vi "Target.vi"() -> ()   [LabVIEW 2018]
uses:
  <vilib>/Platform/TimedLoop/XDataNode/timing_clust.ctl
  <vilib>/Platform/TimedLoop/XDataNode/nitl_modes.ctl
  <vilib>/Platform/TimedLoop/XDataNode/wakeup.ctl
  <vilib>/rvi/eio/common/nirviEmuTemplateMethod_errors.vi
  <vilib>/rvi/Emulation/niFpgaGetClockAttributes.vi
  <vilib>/rvi/Emulation/niFpgaSctlEmulationGetInTimedLoop.vi
  <vilib>/rvi/Emulation/niFpgaEmulationReportErrorSimple.vi
  <vilib>/rvi/Emulation/niFpgaProcessEmulError.vi
  <vilib>/rvi/Emulation/niFpgaCriticalErrorInLSC.vi
  <vilib>/rvi/DataTransferAndStorage/Container/Common/niFpgaContainerGetUniqueNameForEmu.vi
  <vilib>/rvi/Memory/Memory_Emulation/niFpgaMemoryFastEmulationDramWriteAndRequestData.vi
  <vilib>/rvi/Memory/Memory_Emulation/niFpgaMemoryEmulationDramWriteAndRequestData.vi
  <vilib>/rvi/Memory/Memory_Emulation/niFpgaMemoryEmulationDramWriteAndRequestDataApplyByteEnables.vi
  <vilib>/rvi/interface/RandomDataEmulation/niFpgaRandomDataHandleErrors.vi
  <vilib>/eio/EIONode/EIONode.xnode
  <vilib>/Platform/TimedLoop/XDataNode/XDataNode.xnode
  <vilib>/rvi/DataTransferAndStorage/Container/XNode/niFpgaContainer.xnode
  <vilib>/rvi/Memory/Memory_Emulation/niFpgaMemoryEmulationDramRetrieveData.vi
  <vilib>/rvi/interface/RandomDataEmulation/nirviRandomDataFpgaReadWriteTemplate.vi
  <vilib>/Platform/TimedLoop/XDataNode/XDNodeRunTimeDep.lvlib
panel:
  in  "SYNC":bool
  in  "Top(T)/Bot(F)":bool
  in  "SPI_532":u16=532
  in  "SPI_260":u16=260
  in  "W(T)/R(F)":bool
  in  "SPI_258":u16=258
  in  "SPI_256":u16=256
  in  "SPI_257":u16=257
  in  "472":u16=472
  in  "477":u16=477
  in  "478":u16=478
  in  "482":u16=482
  in  "500":u16=500
  in  "503":u16=503
  in  "540":u16=540
  in  "558":u16=558
  in  "559":u16=559
  in  "280":u16=280
  in  "348":u16=348
  in  "351":u16=351
  in  "352":u16=352
  in  "355":u16=355
  in  "357":u16=357
  in  "394":u16=394
  in  "399":u16=399
  in  "400":u16=400
  in  "470":u16=470
  in  "134":u16=134
  in  "140":u16=140
  in  "180":u16=180
  in  "220":u16=220
  in  "222":u16=222
  in  "223":u16=223
  in  "224":u16=224
  in  "225":u16=225
  in  "274":u16=274
  in  "279":u16=279
  in  "75":u16=75
  in  "100":u16=100
  in  "107":u16=107
  in  "109":u16=109
  in  "120":u16=120
  in  "121":u16=121
  in  "124":u16=124
  in  "125":u16=125
  in  "128":u16=128
  in  "130":u16=130
  in  "39":u16=39
  in  "33":u16=33
  in  "30":u16=30
  in  "29":u16=29
  in  "28":u16=28
  in  "26":u16=26
  in  "18":u16=18
  in  "15":u16=15
  in  "12":u16=12
  in  "Управление":bool
  in  "560":u16=560
  in  "12_CLK":u8=12
  in  "DATA_16":u8=16
  in  "6881280":u32=6881280
  in  "Стоп":bool
  out "SPI_OFF":bool
  in  "SPI_IN":bool[](array[boolean])
  out "SPI_OUT":bool[](array[boolean])=[FALSE, FALSE, FALSE, FALSE, FALSE, FALSE, FALSE, FALSE, FALSE, FALSE, FALSE, FALSE, FALSE, FALSE, FALSE, FALSE, FALSE, FALSE, FALSE, FALSE, FALSE, FALSE, FALSE, FALSE, FALSE, FALSE, FALSE, FALSE, FALSE, TRUE, FALSE, TRUE, FALSE, TRUE, FALSE, TRUE, TRUE, TRUE, FALSE, FALSE, TRUE, FALSE, TRUE, TRUE, FALSE, FALSE, FALSE, TRUE, TRUE, TRUE, TRUE, FALSE, FALSE, FALSE, FALSE, FALSE, TRUE, TRUE, TRUE, FALSE, FALSE, FALSE, FALSE, TRUE, TRUE, FALSE, FALSE, FALSE, FALSE, FALSE, FALSE, TRUE, TRUE, FALSE, TRUE, FALSE, TRUE, TRUE, TRUE, FALSE, TRUE, FALSE, TRUE, FALSE, FALSE, FALSE, TRUE, FALSE, FALSE, TRUE, TRUE, FALSE, FALSE, TRUE, TRUE, FALSE, FALSE, FALSE, FALSE, FALSE, FALSE, TRUE, TRUE, TRUE, FALSE, TRUE, TRUE, FALSE, FALSE, TRUE, FALSE, FALSE, FALSE, TRUE, TRUE, FALSE, TRUE, TRUE, FALSE, TRUE, FALSE, FALSE, TRUE, TRUE, TRUE, TRUE, TRUE, TRUE, TRUE, FALSE, TRUE, FALSE, FALSE, TRUE, TRUE, FALSE, FALSE, TRUE, FALSE, FALSE, FALSE, FALSE, TRUE, TRUE, TRUE, FALSE, TRUE, FALSE, FALSE, TRUE, FALSE, TRUE, TRUE, FALSE, TRUE, TRUE, TRUE, FALSE, TRUE, FALSE, TRUE, FALSE, TRUE, TRUE, FALSE, FALSE, TRUE, TRUE, FALSE, TRUE, TRUE, TRUE, TRUE, TRUE, TRUE, TRUE, FALSE, TRUE, TRUE, FALSE, TRUE, FALSE, TRUE, FALSE, TRUE, FALSE, TRUE, FALSE, FALSE, FALSE, FALSE, TRUE, FALSE, FALSE, FALSE, TRUE, FALSE, FALSE, FALSE, TRUE, FALSE, FALSE, TRUE, TRUE, TRUE, TRUE, TRUE, FALSE, FALSE, TRUE, FALSE, FALSE, FALSE, TRUE, TRUE, TRUE, TRUE, FALSE, TRUE, TRUE, TRUE, FALSE, FALSE, TRUE, TRUE, TRUE, TRUE, TRUE, FALSE, TRUE, TRUE, TRUE, FALSE, TRUE, FALSE, FALSE, FALSE, TRUE, FALSE, FALSE, TRUE, FALSE, FALSE, FALSE, FALSE, FALSE, TRUE, TRUE, FALSE, FALSE, TRUE, FALSE, TRUE, FALSE, FALSE, FALSE, FALSE, TRUE, FALSE, FALSE, FALSE, TRUE, FALSE, TRUE, TRUE, FALSE, TRUE, TRUE, FALSE, TRUE, TRUE, TRUE]
  in  "SPI":bool
  in  "SYS_RESET":bool
  in  "Автомат":bool
  out "Записали адресов":u32
  in  "Кадр в память":bool
  in  "Кадр на ПК":bool
  in  "Нач_адр":u32
  in  "Кон_адр":u32=122880
  out "Записали FIFO":bool
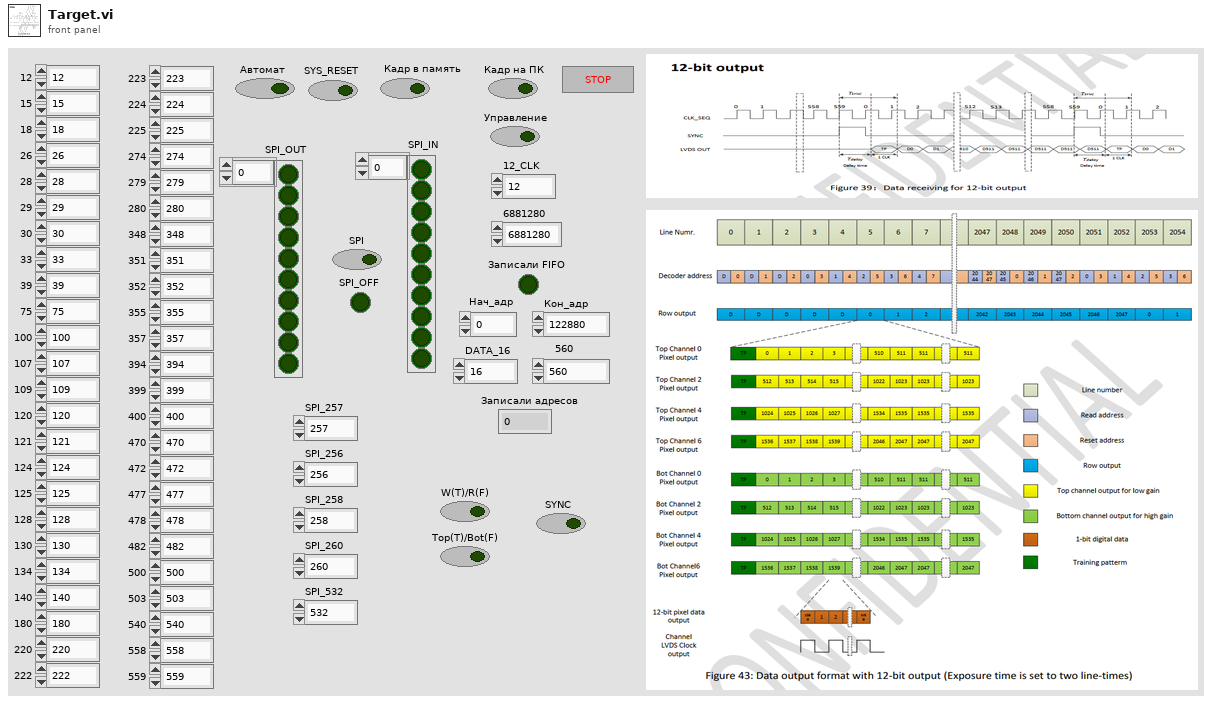
[diagram p1: front panel]
types:
  T1 = typedef "XDNodeRunTimeDep.lvlib/timing_clust.ctl" = cluster{"Expected End [f-1]":u64, "Actual End [f-1]":u64, "Finished Late? [f-1]":bool, "Expected End [i-1]":u64, "Actual End [i-1]":u64, "Finished Late? [i-1]":bool, "Expected Start [i]":u64, "Actual Start [i]":u64, "Expected Start [f]":u64, "Actual Start [f]":u64, "Source Name":string, "Structure Name":string, "Period":i64, "Deadline":i64, "Offset":i64, "Start":i64, "Priority":i32, "Timeout":i32, "Mode":T2, "Wakeup Reason":T3, "Error":errorcluster, "Source Type":string, "Secondary Source Type":string, "Global End Time":u64, "Global Start Time":u64, "Frame Duration":u64, "Iteration Duration":u64, "Assigned CPU":i32, "I/O Scan Engine Mode":u32}
  T2 = typedef "XDNodeRunTimeDep.lvlib/nitl_modes.ctl" = enum32{"No Change", "Process missed periods, maintain original phase", "Discard missed periods, maintain original phase", "Process missed periods, ignore original phase", "Discard missed periods, ignore original phase"}
  T3 = typedef "XDNodeRunTimeDep.lvlib/wakeup.ctl" = enum32{"Normal", "Aborted", "Asynchronous wakeup", "Timing source error", "Timed loop error", "Timeout"}
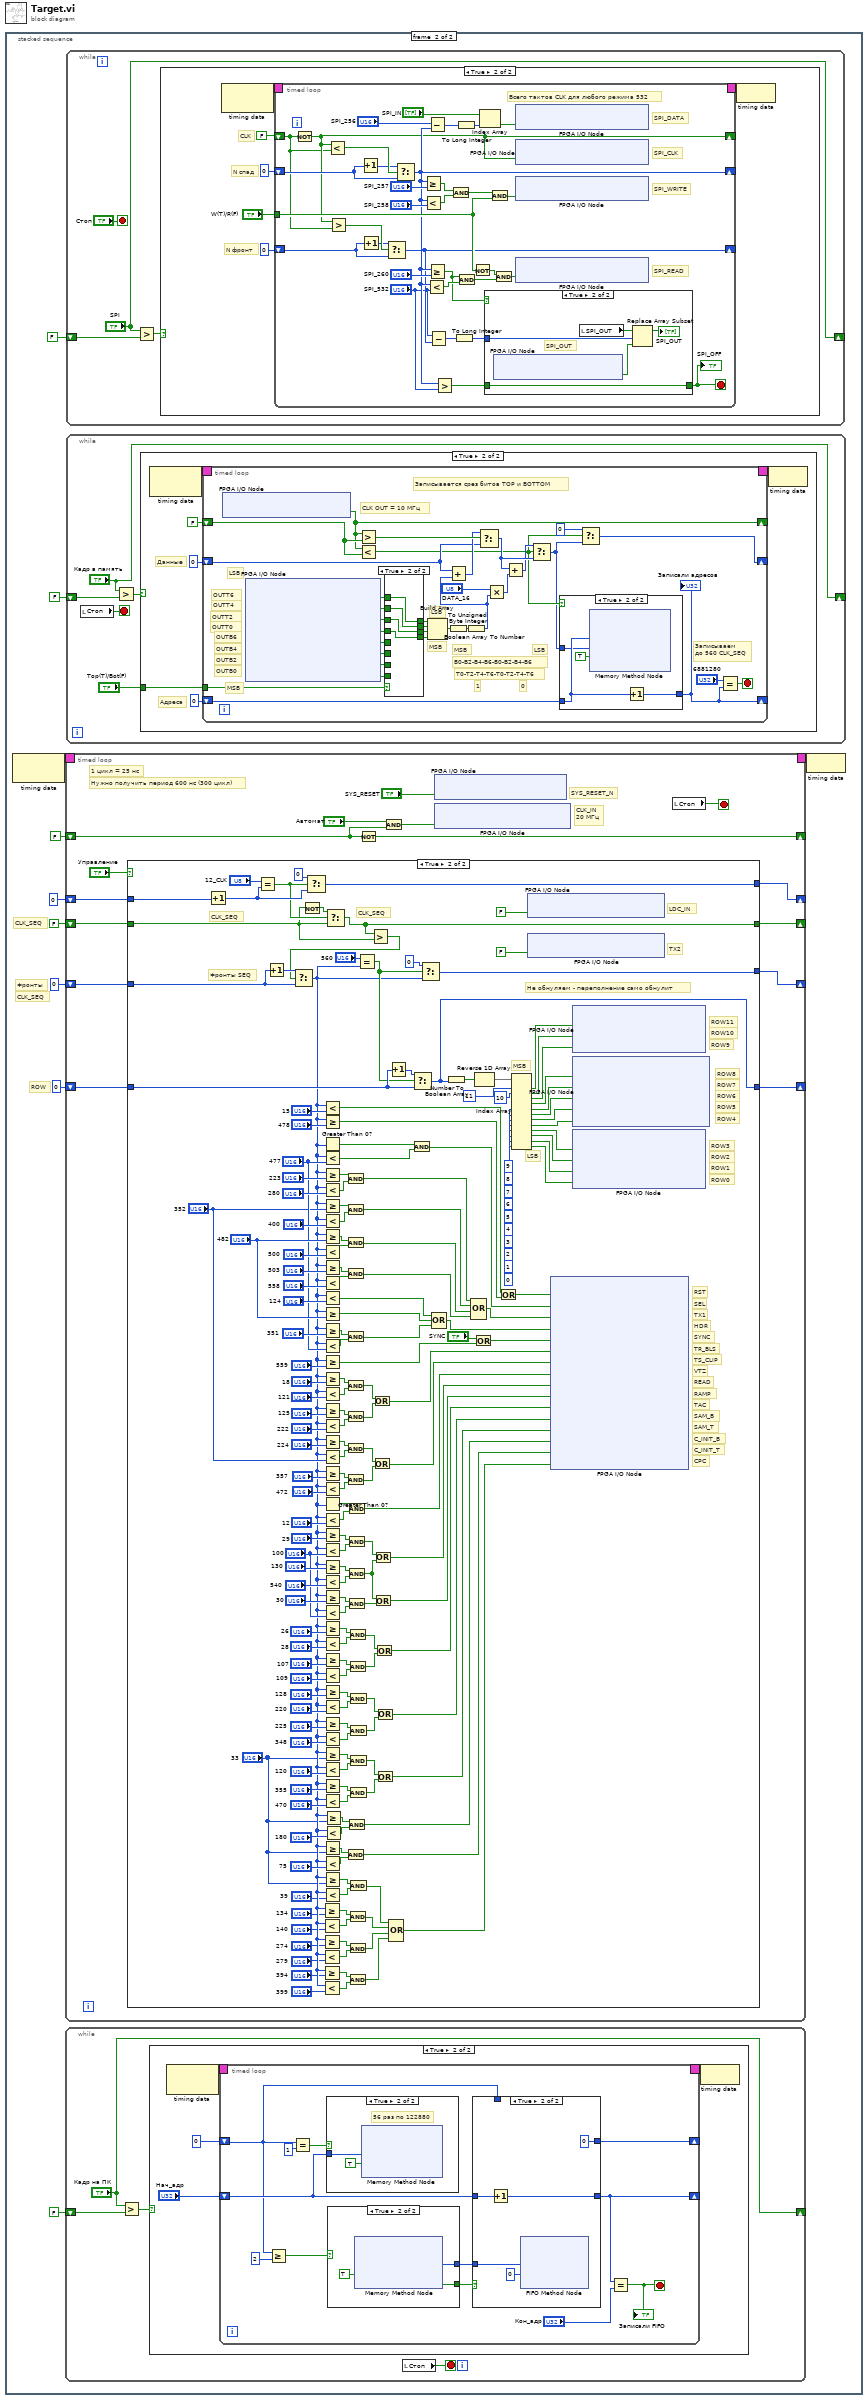
[diagram p0: block diagram]
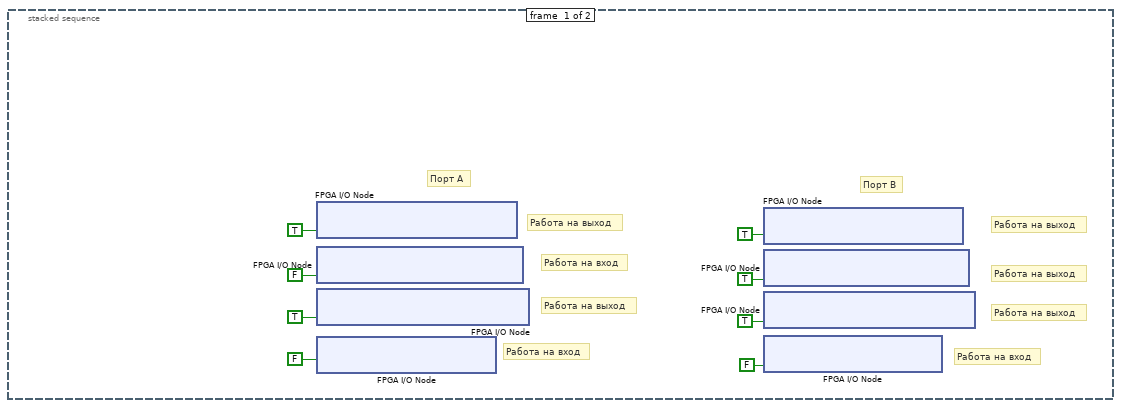
[diagram p2: hidden frame]
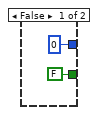
[diagram p6: hidden frame]
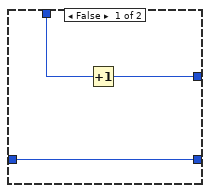
[diagram p8: hidden frame]
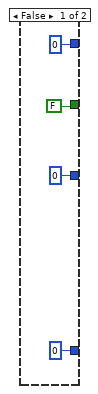
[diagram p12: hidden frame]
diagram:
  n1 = stacked-sequence {
    frame #0 {
      # "Работа на вход"
      # "Работа на вход"
      # "Работа на выход"
      # "Работа на выход"
      # "Работа на выход"
      # "Работа на вход"
      # "Порт В"
      # "Работа на выход"
      # "Порт А"
      # "Работа на выход"
      n2 = xnode "FPGA I/O Node"("IO Module\\DDCA_DIO0-7_WE"=TRUE ("IO Module\\DDCA_DIO0-7_WE")) -> ()  [unwired: 1 in, 1 out]
      n3 = xnode "FPGA I/O Node"("IO Module\\DDCA_DIO8-15_WE"=FALSE ("IO Module\\DDCA_DIO8-15_WE")) -> ()  [unwired: 1 in, 1 out]
      n4 = xnode "FPGA I/O Node"("IO Module\\DDCA_DIO16-23_WE"=TRUE ("IO Module\\DDCA_DIO16-23_WE")) -> ()  [unwired: 1 in, 1 out]
      n5 = xnode "FPGA I/O Node"("IO Module\\DDCA_PFI_WE"=FALSE ("IO Module\\DDCA_DIO16-23_WE")) -> ()  [unwired: 1 in, 1 out]
      n6 = xnode "FPGA I/O Node"("IO Module\\DDCB_DIO0-7_WE"=TRUE ("IO Module\\DDCA_DIO0-7_WE")) -> ()  [unwired: 1 in, 1 out]
      n7 = xnode "FPGA I/O Node"("IO Module\\DDCB_DIO8-15_WE"=TRUE ("IO Module\\DDCA_DIO8-15_WE")) -> ()  [unwired: 1 in, 1 out]
      n8 = xnode "FPGA I/O Node"("IO Module\\DDCB_DIO16-23_WE"=TRUE ("IO Module\\DDCA_DIO16-23_WE")) -> ()  [unwired: 1 in, 1 out]
      n9 = xnode "FPGA I/O Node"("IO Module\\DDCB_PFI_WE"=FALSE ("IO Module\\DDCA_DIO16-23_WE")) -> ()  [unwired: 1 in, 1 out]
    }
    frame #1 {
      # "CLK_SEQ"
      # "Фронты"
      # "CLK_SEQ"
      # "ROW"
      n10 = node-c288() -> (w18:T1)  [unwired: 1 in]
      n11 = timed-loop {
        timing: w18 -> [_]
        timing-out: [_] -> w17
        shift-right: [w184] -> _
        shift-left: FALSE -> [w179]
        shift-right: [w181] -> _
        shift-left: u16 0 -> [w182]
        shift-right: [w178] -> _
        shift-left: u8 0 -> [w180]
        shift-right: [w176] -> _
        shift-left: u16 0 -> [w177]
        shift-right: [w172] -> _
        shift-left: FALSE -> [w173]
        stop <- w183 stop-if-true
        # "Нужно получить период 600 нс (300 цикл)"
        # "1 цикл = 25 нс"
        # "SYS_RESET_N"
        # "CLK_IN\n20 МГц"
        n12 = case shown="True" "Управление" {
          tunnel: w182 -> [_ w369]
          tunnel: [u16 0 w368] -> w181
          tunnel: w180 -> [_ w367]
          tunnel: [u8 0 w364] -> w178
          tunnel: w177 -> [_ w362]
          tunnel: [u16 0 w357] -> w176
          tunnel: w173 -> [_ w351]
          tunnel: [FALSE w352] -> w172
          frame False {
          }
          frame True {
            # "CPC"
            # "C_INIT_T"
            # "C_INIT_B"
            # "SAM_T"
            # "SAM_B"
            # "TAC"
            # "RAMP"
            # "READ"
            # "VTZ"
            # "TS_CLIP"
            # "TR_BLS"
            # "SYNC"
            # "HDR"
            # "TX1"
            # "SEL"
            # "RST"
            # "TX2"
            # "LDC_IN"
            # "CLK_SEQ"
            # "CLK_SEQ"
            # "Не обнуляем - переполнение само обнулит"
            # "Фронты SEQ"
            # "LSB"
            # "MSB"
            # "ROW0"
            # "ROW1"
            # "ROW2"
            # "ROW3"
            # "ROW4"
            # "ROW5"
            # "ROW6"
            # "ROW7"
            # "ROW8"
            # "ROW9"
            # "ROW10"
            # "ROW11"
            n13 = Increment(x=w367) -> (x+1=w365:u8)
            n14 = Equal?(x="12_CLK", y=w365) -> (x = y?=w354:bool)
            n15 = Increment(x=w362) -> (x+1=w361:u16)
            n16 = Not(x=w351) -> (.not. x?=w353:bool)
            n17 = Select(t=u8 0, s=w354, f=w365) -> (s? t:f=w364:u8)
            n18 = Select(t=w353, s=w354, f=w351) -> (s? t:f=w352:bool)
            n19 = Greater?(x=w352, y=w351) -> (0:w350:bool)
            n20 = Select(t=w361, s=w350, f=w362) -> (s? t:f=w215:u16)
            n21 = Greater Or Equal?(x=w215, y="134") -> (x >= y?=w226:bool)
            n22 = Less?(x=w215, y="140") -> (x < y?=w225:bool)
            n23 = Greater Or Equal?(x=w215, y="274") -> (x >= y?=w223:bool)
            n24 = Less?(x=w215, y="279") -> (x < y?=w224:bool)
            n25 = Greater Or Equal?(x=w215, y="394") -> (x >= y?=w222:bool)
            n26 = Less?(x=w215, y="399") -> (x < y?=w221:bool)
            n27 = Less?(x=w215, y="15") -> (x < y?=w346:bool)
            n28 = Greater Or Equal?(x=w215, y="478") -> (x >= y?=w345:bool)
            n29 = Greater Than 0?(x=w215) -> (x > 0?=w342:bool)
            n30 = Less?(x=w215, y="477") -> (x < y?=w341:bool)
            n31 = Greater Or Equal?(x=w215, y="223") -> (x >= y?=w338:bool)
            n32 = Less?(x=w215, y="280") -> (x < y?=w337:bool)
            n33 = Greater Or Equal?(x=w215, y="352") -> (x >= y?=w333:bool)
            n34 = Less?(x=w215, y="400") -> (x < y?=w334:bool)
            n35 = Greater Or Equal?(x=w215, y="482") -> (x >= y?=w330:bool)
            n36 = Less?(x=w215, y="500") -> (x < y?=w329:bool)
            n37 = Greater Or Equal?(x=w215, y="503") -> (x >= y?=w327:bool)
            n38 = Less?(x=w215, y="558") -> (x < y?=w328:bool)
            n39 = Less?(x=w215, y="124") -> (x < y?=w319:bool)
            n40 = Greater Or Equal?(x=w215, y="482") -> (x >= y?=w315:bool)
            n41 = Greater Or Equal?(x=w215, y="351") -> (x >= y?=w318:bool)
            n42 = Less?(x=w215, y="477") -> (x < y?=w317:bool)
            n43 = Greater Or Equal?(x=w215, y="559") -> (x >= y?=w204:bool)
            n44 = Greater Or Equal?(x=w215, y="18") -> (x >= y?=w310:bool)
            n45 = Less?(x=w215, y="121") -> (x < y?=w309:bool)
            n46 = Greater Or Equal?(x=w215, y="125") -> (x >= y?=w308:bool)
            n47 = Less?(x=w215, y="222") -> (x < y?=w307:bool)
            n48 = Greater Or Equal?(x=w215, y="224") -> (x >= y?=w294:bool)
            n49 = Less?(x=w215, y="352") -> (x < y?=w295:bool)
            n50 = Greater Or Equal?(x=w215, y="357") -> (x >= y?=w296:bool)
            n51 = Less?(x=w215, y="472") -> (x < y?=w297:bool)
            n52 = Greater Than 0?(x=w215) -> (x > 0?=w287:bool)
            n53 = Less?(x=w215, y="12") -> (x < y?=w288:bool)
            n54 = Greater Or Equal?(x=w215, y="29") -> (x >= y?=w284:bool)
            n55 = Less?(x=w215, y="100") -> (x < y?=w283:bool)
            n56 = Greater Or Equal?(x=w215, y="130") -> (x >= y?=w282:bool)
            n57 = Less?(x=w215, y="540") -> (x < y?=w281:bool)
            n58 = Greater Or Equal?(x=w215, y="30") -> (x >= y?=w278:bool)
            n59 = Less?(x=w215, y="100") -> (x < y?=w279:bool)
            n60 = Greater Or Equal?(x=w215, y="26") -> (x >= y?=w268:bool)
            n61 = Less?(x=w215, y="28") -> (x < y?=w267:bool)
            n62 = Greater Or Equal?(x=w215, y="107") -> (x >= y?=w266:bool)
            n63 = Less?(x=w215, y="109") -> (x < y?=w265:bool)
            n64 = Greater Or Equal?(x=w215, y="128") -> (x >= y?=w252:bool)
            n65 = Less?(x=w215, y="220") -> (x < y?=w253:bool)
            n66 = Greater Or Equal?(x=w215, y="225") -> (x >= y?=w254:bool)
            n67 = Less?(x=w215, y="348") -> (x < y?=w255:bool)
            n68 = Greater Or Equal?(x=w215, y="33") -> (x >= y?=w246:bool)
            n69 = Less?(x=w215, y="120") -> (x < y?=w245:bool)
            n70 = Greater Or Equal?(x=w215, y="355") -> (x >= y?=w244:bool)
            n71 = Less?(x=w215, y="470") -> (x < y?=w243:bool)
            n72 = Greater Or Equal?(x=w215, y="33") -> (x >= y?=w232:bool)
            n73 = Less?(x=w215, y="75") -> (x < y?=w231:bool)
            n74 = Greater Or Equal?(x=w215, y="33") -> (x >= y?=w227:bool)
            n75 = Less?(x=w215, y="39") -> (x < y?=w228:bool)
            n76 = Greater Or Equal?(x=w215, y="33") -> (x >= y?=w235:bool)
            n77 = Less?(x=w215, y="180") -> (x < y?=w236:bool)
            n78 = And(x=w338, y=w337) -> (x .and. y?=w335:bool)
            n79 = And(x=w333, y=w334) -> (x .and. y?=w331:bool)
            n80 = And(x=w330, y=w329) -> (x .and. y?=w323:bool)
            n81 = And(x=w327, y=w328) -> (x .and. y?=w322:bool)
            n82 = And(x=w318, y=w317) -> (x .and. y?=w313:bool)
            n83 = And(x=w310, y=w309) -> (x .and. y?=w306:bool)
            n84 = And(x=w308, y=w307) -> (x .and. y?=w305:bool)
            n85 = And(x=w294, y=w295) -> (x .and. y?=w298:bool)
            n86 = And(x=w296, y=w297) -> (x .and. y?=w299:bool)
            n87 = And(x=w232, y=w231) -> (x .and. y?=w229:bool)
            n88 = And(x=w287, y=w288) -> (x .and. y?=w285:bool)
            n89 = And(x=w284, y=w283) -> (x .and. y?=w280:bool)
            n90 = And(x=w282, y=w281) -> (x .and. y?=w271:bool)
            n91 = And(x=w235, y=w236) -> (x .and. y?=w234:bool)
            n92 = And(x=w278, y=w279) -> (x .and. y?=w272:bool)
            n93 = And(x=w268, y=w267) -> (x .and. y?=w264:bool)
            n94 = And(x=w266, y=w265) -> (x .and. y?=w263:bool)
            n95 = And(x=w226, y=w225) -> (x .and. y?=w219:bool)
            n96 = And(x=w223, y=w224) -> (x .and. y?=w218:bool)
            n97 = And(x=w222, y=w221) -> (x .and. y?=w217:bool)
            n98 = And(x=w252, y=w253) -> (x .and. y?=w256:bool)
            n99 = And(x=w254, y=w255) -> (x .and. y?=w257:bool)
            n100 = And(x=w246, y=w245) -> (x .and. y?=w242:bool)
            n101 = And(x=w244, y=w243) -> (x .and. y?=w241:bool)
            n102 = And(x=w227, y=w228) -> (x .and. y?=w220:bool)
            n103 = Equal?(x="560", y=w215) -> (x = y?=w355:bool)
            n104 = Or(x=w306, y=w305) -> (x .or. y?=w304:bool)
            n105 = Or(x=w298, y=w299) -> (x .or. y?=w289:bool)
            n106 = Or(x=w280, y=w271) -> (x .or. y?=w277:bool)
            n107 = Or(x=w271, y=w272) -> (x .or. y?=w276:bool)
            n108 = Or(x=w264, y=w263) -> (x .or. y?=w262:bool)
            n109 = Or(x=w256, y=w257) -> (x .or. y?=w247:bool)
            n110 = Or(x=w242, y=w241) -> (x .or. y?=w237:bool)
            n111 = Increment(x=w369) -> (x+1=w370:u16)
            n112 = Compound Arithmetic op=OR(w220, w219, w218, w217) -> (w216:bool)
            n113 = And(x=w342, y=w341) -> (x .and. y?=w340:bool)
            n114 = Select(t=w370, s=w355, f=w369) -> (s? t:f=w368:u16)
            n115 = Select(t=u16 0, s=w355, f=w215) -> (s? t:f=w357:u16)
            n116 = Compound Arithmetic op=OR(w319, w315, w313) -> (w321:bool)
            n117 = Number To Boolean Array(number=w368) -> (Boolean array=w360:bool[])
            n118 = Compound Arithmetic op=OR(w335, w331, w323, w322) -> (w206:bool)
            n119 = Or(x="SYNC", y=w204) -> (x .or. y?=w205:bool)
            n120 = Reverse 1D Array(array=w360) -> (reversed array=w359:bool[])
            n121 = Or(x=w346, y=w345) -> (x .or. y?=w344:bool)
            n122 = Index Array(array=w359, index #1=11 ("index"), index #2=10 ("index"), index #3=9 ("index"), index #4=8 ("index"), index #5=7 ("index"), index #6=6 ("index"), index #7=5 ("index"), index #8=4 ("index"), index #9=3 ("index"), index #10=2 ("index"), index #11=1 ("index"), index #12=0 ("index")) -> (element #1=w382:bool, element #2=w381:bool, element #3=w380:bool, element #4=w379:bool, element #5=w378:bool, element #6=w377:bool, element #7=w376:bool, element #8=w375:bool, element #9=w374:bool, element #10=w373:bool, element #11=w372:bool, element #12=w371:bool)
            n123 = xnode "FPGA I/O Node"("IO Module\\DDCB_DIO11_Write"=FALSE ("IO Module\\DDCB_DIO12_Write")) -> ()  [unwired: 1 in, 1 out]
            n124 = xnode "FPGA I/O Node"("IO Module\\DDCA_DIO17_Write"=FALSE ("IO Module\\DDCB_DIO12_Write")) -> ()  [unwired: 1 in, 1 out]
            n125 = xnode "FPGA I/O Node"("IO Module\\DDCB_DIO3_Write"=w344, "IO Module\\DDCB_DIO5_Write"=w340, "IO Module\\DDCA_DIO18_Write"=w206, "IO Module\\DDCA_DIO6_Write"=w321, "IO Module\\DDCB_DIO16_Write"=w205, "IO Module\\DDCB_DIO13_Write"=w304, "IO Module\\DDCB_DIO14_Write"=w289, "IO Module\\DDCB_DIO8_Write"=w285, "IO Module\\DDCB_DIO22_Write"=w277, "IO Module\\DDCB_DIO15_Write"=w276, "IO Module\\DDCB_DIO10_Write"=w262, "IO Module\\DDCB_DIO21_Write"=w247, "IO Module\\DDCB_DIO19_Write"=w237, "IO Module\\DDCB_DIO18_Write"=w234, "IO Module\\DDCB_DIO17_Write"=w229, "IO Module\\DDCB_DIO9_Write"=w216) -> ()  [unwired: 16 in, 16 out]
            n126 = xnode "FPGA I/O Node"("IO Module\\DDCA_DIO1_Write"=w382, "IO Module\\DDCA_DIO2_Write"=w381, "IO Module\\DDCA_DIO7_Write"=w380) -> ()  [unwired: 3 in, 3 out]
            n127 = xnode "FPGA I/O Node"("IO Module\\DDCA_DIO16_Write"=w379, "IO Module\\DDCA_DIO19_Write"=w378, "IO Module\\DDCA_DIO20_Write"=w377, "IO Module\\DDCA_DIO21_Write"=w376, "IO Module\\DDCA_DIO22_Write"=w375) -> ()  [unwired: 5 in, 5 out]
            n128 = xnode "FPGA I/O Node"("IO Module\\DDCB_DIO0_Write"=w374, "IO Module\\DDCB_DIO1_Write"=w373, "IO Module\\DDCB_DIO2_Write"=w372, "IO Module\\DDCB_DIO4_Write"=w371) -> ()  [unwired: 4 in, 4 out]
          }
        }
        n129 = Not(x=w179) -> (.not. x?=w184:bool)
        n130 = And(x="Автомат", y=w179) -> (x .and. y?=w185:bool)
        n131 = xnode "FPGA I/O Node"("IO Module\\DDCB_DIO7_Write"="SYS_RESET") -> ()  [unwired: 1 in, 1 out]
        n132 = xnode "FPGA I/O Node"("IO Module\\DDCB_DIO12_Write"=w185) -> ()  [unwired: 1 in, 1 out]
        n133 = local read "Стоп"() -> (w183:bool)
      }
      n134 = while {
        shift-right: ["Кадр на ПК"] -> _
        shift-left: FALSE ("Кадр на ПК") -> [w73]
        stop <- w75 stop-if-true
        n135 = Greater?(x="Кадр на ПК", y=w73) -> (0:w74:bool)
        n136 = case shown="True" w74 {
          frame False {
          }
          frame True {
            n137 = node-c288() -> (w79:T1)  [unwired: 1 in]
            n138 = timed-loop {
              shift-right: [w90] -> _
              shift-left: "Нач_адр" -> [w84]
              timing: w79 -> [_]
              timing-out: [_] -> w78
              shift-right: [w82] -> _
              shift-left: u8 0 -> [w83]
              stop <- w91 stop-if-true
              n139 = Greater Or Equal?(x=w83, y=u8 2 ("2")) -> (x >= y?=w85:bool)
              n140 = Equal?(x=w83, y=u8 1 ("1")) -> (x = y?=w88:bool)
              n141 = case shown="True" w88 {
                tunnel: w84 -> [_ w97]
                frame False {
                }
                frame True {
                  # "56 раз по 122880"
                  n142 = xnode ("Memory Method Node")("Address"=w97, "Input Valid"=TRUE) -> ()  [unwired: 1 in, 2 out]
                }
              }
              n143 = case shown="True" w85 {
                tunnel: [u8 0 ("Data") w95] -> w89
                tunnel: [FALSE ("Output Valid") w96] -> w80
                frame False {
                }
                frame True {
                  n144 = xnode ("Memory Method Node")("Ready for Output"=TRUE ("Ready For Output")) -> ("Data"=w95:u8, "Output Valid"=w96:bool)  [unwired: 1 in, 1 out]
                }
              }
              n145 = case shown="True" w80 {
                tunnel: [w99 w106] -> w90
                tunnel: w89 -> [_ w102]
                tunnel: w84 -> [w99 w105]
                tunnel: w83 -> [w101 _]
                tunnel: [w100 u8 0] -> w82
                frame False {
                  n146 = Increment(x=w101) -> (x+1=w100:u8)
                }
                frame True {
                  n147 = Increment(x=w105) -> (x+1=w106:u32)
                  n148 = xnode ("FIFO Method Node")("Element"=w102, "Timeout"=0) -> ()  [unwired: 1 in, 2 out]
                }
              }
              n149 = Equal?(x=w90, y="Кон_адр") -> (x = y?=w91:bool)
              "Записали FIFO" <- w91
            }
            n150 = node-c288(w78) -> ()
          }
        }
        n151 = local read "Стоп"() -> (w75:bool)
      }
      n152 = while {
        shift-right: ["SPI"] -> _
        shift-left: FALSE ("SPI") -> [w20]
        stop <- "Стоп" stop-if-true
        n153 = Greater?(x="SPI", y=w20) -> (0:w21:bool)
        n154 = case shown="True" w21 {
          frame False {
          }
          frame True {
            # "N фронт"
            # "N спад"
            # "CLK"
            n155 = node-c288() -> (w28:T1)  [unwired: 1 in]
            n156 = timed-loop {
              timing: w28 -> [_]
              timing-out: [_] -> w27
              shift-right: [w39] -> _
              shift-left: FALSE -> [w38]
              shift-right: [w41] -> _
              shift-left: u16 0 -> [w59]
              tunnel: "W(T)/R(F)" -> [w46]
              shift-right: [w34] -> _
              shift-left: u16 0 -> [w35]
              stop <- w55 stop-if-true
              # "Всего тактов CLK для любого режима 532"
              # "SPI_READ"
              # "SPI_WRITE"
              # "SPI_DATA"
              # "SPI_CLK"
              n157 = Not(x=w38) -> (.not. x?=w39:bool)
              n158 = Less?(x=w39, y=w38) -> (x < y?=w61:bool)
              n159 = Greater?(x=w39, y=w38) -> (0:w37:bool)
              n160 = Increment(x=w59) -> (x+1=w60:u16)
              n161 = Increment(x=w35) -> (x+1=w36:u16)
              n162 = Select(t=w36, s=w37, f=w35) -> (s? t:f=w34:u16)
              n163 = Select(t=w60, s=w61, f=w59) -> (s? t:f=w41:u16)
              n164 = Greater Or Equal?(x=w41, y="SPI_257") -> (x >= y?=w57:bool)
              n165 = Less?(x=w41, y="SPI_258") -> (x < y?=w58:bool)
              n166 = Less?(x=w41, y="SPI_532") -> (x < y?=w45:bool)
              n167 = Subtract(x="SPI_256", y=w41) -> (x-y=w31:u16)
              n168 = Greater Or Equal?(x=w41, y="SPI_260") -> (x >= y?=w43:bool)
              n169 = Subtract(x="SPI_532", y=w34) -> (x-y=w30:u16)
              n170 = Greater?(x=w41, y="SPI_532") -> (0:w56:bool)
              n171 = And(x=w57, y=w58) -> (x .and. y?=w49:bool)
              n172 = To Long Integer(number=w30) -> (32bit integer=w29:i32)
              n173 = To Long Integer(number=w31) -> (32bit integer=w32:i32)
              n174 = And(x=w43, y=w45) -> (x .and. y?=w44:bool)
              n175 = Not(x=w46) -> (.not. x?=w47:bool)
              n176 = Index Array(array="SPI_IN", index=w32) -> (element=w53:bool)
              n177 = case shown="True" w43 {
                tunnel: [w62 w65] -> w55
                tunnel: w56 -> [w62 w65]
                tunnel: w29 -> [_ w64]
                frame False {
                }
                frame True {
                  # "SPI_OUT"
                  n178 = xnode "FPGA I/O Node"() -> ("IO Module\\DDCA_PFI1_Read"=w63:bool)  [unwired: 1 in, 1 out]
                  n179 = local read "SPI_OUT"() -> (w66:bool[])
                  n180 = Replace Array Subset(array=w66, new element=w63, index=w64) -> (→"SPI_OUT":bool[])
                }
              }
              "SPI_OFF" <- w55
              n181 = And(x=w49, y=w46) -> (x .and. y?=w50:bool)
              n182 = And(x=w47, y=w44) -> (x .and. y?=w48:bool)
              n183 = xnode "FPGA I/O Node"("IO Module\\DDCA_DIO3_Write"=w53) -> ()  [unwired: 1 in, 1 out]
              n184 = xnode "FPGA I/O Node"("IO Module\\DDCA_DIO4_Write"=w39) -> ()  [unwired: 1 in, 1 out]
              n185 = xnode "FPGA I/O Node"("IO Module\\DDCA_DIO0_Write"=w50) -> ()  [unwired: 1 in, 1 out]
              n186 = xnode "FPGA I/O Node"("IO Module\\DDCA_DIO5_Write"=w48) -> ()  [unwired: 1 in, 1 out]
            }
            n187 = node-c288(w27) -> ()
          }
        }
      }
      n188 = while {
        shift-right: ["Кадр в память"] -> _
        shift-left: FALSE -> [w114]
        stop <- w115 stop-if-true
        n189 = local read "Стоп"() -> (w115:bool)
        n190 = Greater?(x="Кадр в память", y=w114) -> (0:w113:bool)
        n191 = case shown="True" w113 {
          tunnel: "Top(T)/Bot(F)" -> [_ w116]
          frame False {
          }
          frame True {
            # "Данные"
            # "Адреса"
            n192 = node-c288() -> (w121:T1)  [unwired: 1 in]
            n193 = timed-loop {
              timing: w121 -> [_]
              timing-out: [_] -> w120
              shift-right: [w141] -> _
              shift-left: u32 0 -> [w154]
              shift-right: [w152] -> _
              shift-left: FALSE -> [w153]
              shift-right: [w135] -> _
              shift-left: u8 0 -> [w147]
              tunnel: w116 -> [w134]
              stop <- w139 stop-if-true
              # "Записываем\nдо 560 CLK_SEQ"
              # "T0-T2-T4-T6-T0-T2-T4-T6"
              # "LSB"
              # "MSB"
              # "0"
              # "MSB"
              # "1"
              # "LSB"
              # "B0-B2-B4-B6-B0-B2-B4-B6"
              # "OUTB0"
              # "OUTB2"
              # "OUTB4"
              # "OUTB6"
              # "OUTT2"
              # "OUTT0"
              # "OUTT4"
              # "OUTT6"
              # "LSB"
              # "MSB"
              # "CLK OUT = 10 МГц"
              # "Записывается срез битов TOP и BOTTOM"
              n194 = xnode "FPGA I/O Node"() -> ("IO Module\\DDCB_PFI1_Read"=w152:bool)  [unwired: 1 in, 1 out]
              n195 = xnode "FPGA I/O Node"() -> ("IO Module\\DDCA_DIO8_Read"=w133:bool, "IO Module\\DDCA_DIO9_Read"=w132:bool, "IO Module\\DDCA_DIO11_Read"=w131:bool, "IO Module\\DDCA_DIO10_Read"=w130:bool, "IO Module\\DDCA_DIO12_Read"=w125:bool, "IO Module\\DDCA_DIO13_Read"=w124:bool, "IO Module\\DDCA_DIO14_Read"=w123:bool, "IO Module\\DDCA_DIO15_Read"=w122:bool)  [unwired: 8 in, 8 out]
              n196 = Greater?(x=w152, y=w153) -> (0:w150:bool)
              n197 = Less?(x=w152, y=w153) -> (x < y?=w138:bool)
              n198 = case shown="True" w134 {
                tunnel: w133 -> [_ w162]
                tunnel: w132 -> [_ w161]
                tunnel: w131 -> [_ w160]
                tunnel: w130 -> [_ w159]
                tunnel: [w158 w162] -> w129
                tunnel: [w157 w161] -> w128
                tunnel: [w156 w160] -> w127
                tunnel: [w155 w159] -> w126
                tunnel: w125 -> [w158 _]
                tunnel: w124 -> [w157 _]
                tunnel: w123 -> [w156 _]
                tunnel: w122 -> [w155 _]
                frame False {
                }
                frame True {
                }
              }
              n199 = Build Array(w129, w128, w127, w126) -> (w151:bool[])
              n200 = Boolean Array To Number(Boolean array=w151) -> (number=w149:u8)
              n201 = To Unsigned Byte Integer(number=w149) -> (unsigned 8bit integer=w143:u8)
              n202 = Add(x=w147, y=w143) -> (x+y=w148:u8)
              n203 = Select(t=w148, s=w150, f=w147) -> (s? t:f=w146:u8)
              n204 = Multiply(x="DATA_16", y=w143) -> (x*y=w144:u8)
              n205 = Add(x=w146, y=w144) -> (x+y=w145:u8)
              n206 = Select(t=w145, s=w138, f=w146) -> (s? t:f=w137:u8)
              n207 = case shown="True" w138 {
                tunnel: w154 -> [w163 w167]
                tunnel: [w163 w166] -> w141
                tunnel: w137 -> [_ w164]
                frame False {
                }
                frame True {
                  n208 = xnode ("Memory Method Node")("Address"=w167, "Data"=w164, "Input Valid"=TRUE) -> ()  [unwired: 1 in, 2 out]
                  n209 = Increment(x=w167) -> (x+1=w166:u32)
                }
              }
              "Записали адресов" <- w141
              n210 = Select(t=u8 0, s=w138, f=w137) -> (s? t:f=w135:u8)
              n211 = Equal?(x="6881280", y=w141) -> (x = y?=w139:bool)
            }
            n212 = node-c288(w120) -> ()
          }
        }
      }
      n213 = node-c288(w17) -> ()
    }
  }
